vi "tm424_triggermodes.vi"() -> ()   [LabVIEW 2021]
panel:
  in  "Times":i32=1
  in  "Active":i32(ring)=1 items=["Edge"=1, "Level"=2, "Sync Readout"=3, "Point"=4]
  in  "External Options":cluster{"Polarity":i32, "Delay":dbl}={"Polarity"=1, "Delay"=0.0} {"Polarity" items=["Negative"=1, "Positive"=2]}
  in  "Source":i32(ring)=1 items=["Internal"=1, "External"=2, "Software"=3, "Master Pulse"=4]
  out "Timestamp":dbl
  out "Image":u16[][](graph)
  out "Frames Per Second":dbl
  in  "Quit":bool
  out "Error Out":errorcluster {"code" format="%.0x"}
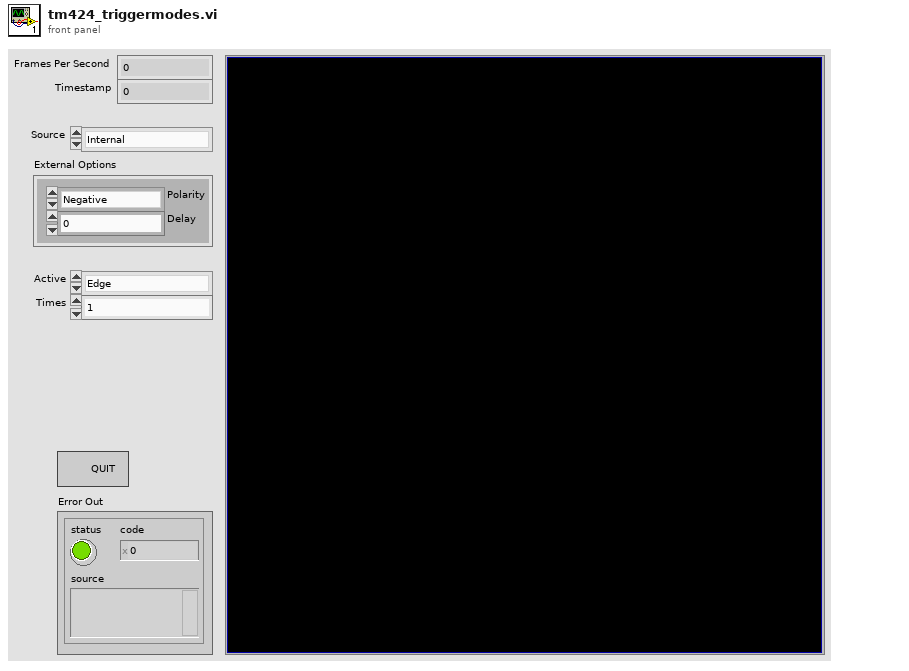
[diagram p1: front panel]
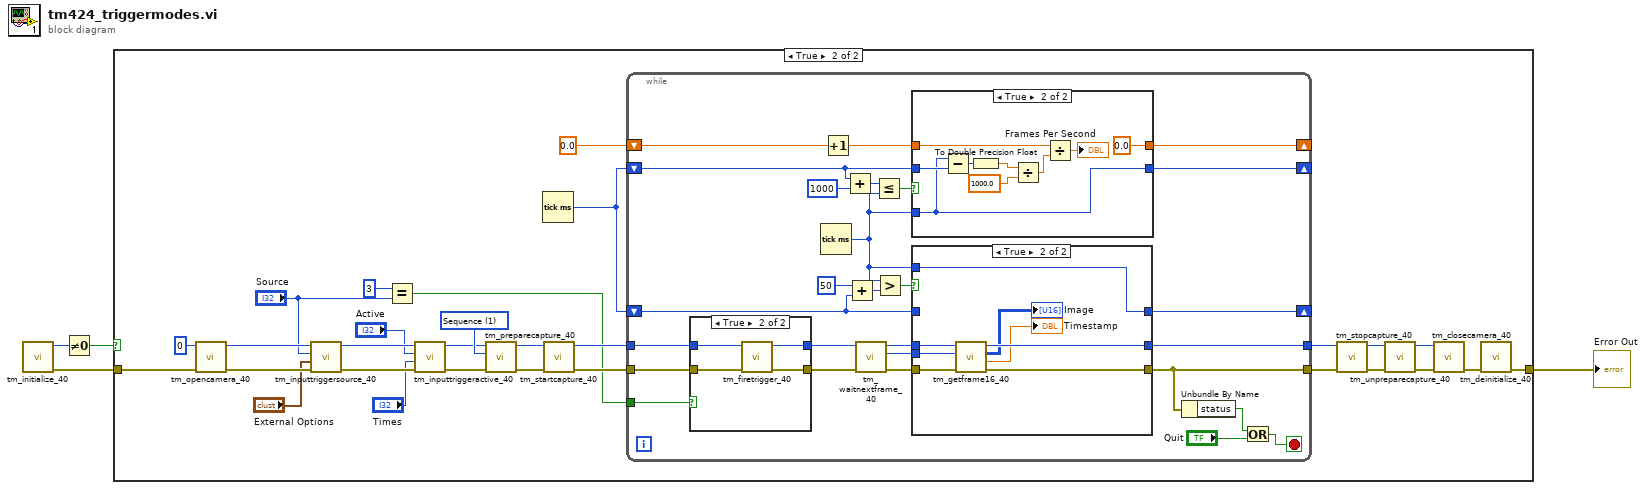
[diagram p0: block diagram]
diagram:
  n1 = call <userlib>:"tm_initialize_40.vi"() -> ("error out"=w2:errorcluster, "Number Of Cameras"=w3:u32)  [unwired: 8 in, 2 out]
  n2 = Not Equal To 0?(x=w3) -> (x != 0?=w4:bool)
  n3 = case shown="True" w4 {
    tunnel: w2 -> [w5 w34]
    tunnel: [w5 w18] -> w1
    frame False {
    }
    frame True {
      w24 = 1 items=["Snap", "Sequence"] ("Capture mode")
      n4 = call <userlib>:"tm_opencamera_40.vi"("error in (no error)"=w34, "Camera Index"=u32 0) -> ("error out"=w17:errorcluster, "Handle out"=w16:u32)  [unwired: 7 in, 1 out]
      n5 = call <userlib>:"tm_inputtriggersource_40.vi"("error in (no error)"=w17, "External Options"="External Options", "Source"="Source", "Handle in"=w16) -> ("error out"=w14:errorcluster, "Handle out"=w15:u32)  [unwired: 6 in]
      n6 = Equal?(x=3, y="Source") -> (x = y?=w6:bool)
      n7 = call <userlib>:"tm_inputtriggeractive_40.vi"("error in (no error)"=w14, "Times"="Times", "Active"="Active", "Handle in"=w15) -> ("error out"=w9:errorcluster, "Handle out"=w10:u32)  [unwired: 6 in]
      n8 = call <userlib>:"tm_preparecapture_40.vi"("error in (no error)"=w9, "Capture mode"=w24, "Handle in"=w10) -> ("error out"=w22:errorcluster, "Handle out"=w23:u32)  [unwired: 5 in, 2 out]
      n9 = Tick Count (ms)() -> (millisecond timer value=w20:u32)
      n10 = call <userlib>:"tm_startcapture_40.vi"("error in (no error)"=w22, "Handle in"=w23) -> ("error out"=w25:errorcluster, "Handle out"=w26:u32)  [unwired: 8 in]
      n11 = while {
        tunnel: [w42] -> w29
        tunnel: [w43] -> w30
        tunnel: w26 -> [w38]
        tunnel: w25 -> [w39]
        shift-right: [w58] -> _
        shift-left: w20 -> [w55]
        shift-right: [w59] -> _
        shift-left: 0.0 -> [w52]
        shift-right: [w41] -> _
        shift-left: w20 -> [w44]
        tunnel: w6 -> [w35]
        stop <- w40 stop-if-true
        n12 = case shown="True" w35 {
          tunnel: w39 -> [w62 w66]
          tunnel: w38 -> [w63 w67]
          tunnel: [w62 w65] -> w36
          tunnel: [w63 w64] -> w37
          frame False {
          }
          frame True {
            n13 = call <userlib>:"tm_firetrigger_40.vi"("error in (no error)"=w66, "Handle in"=w67) -> ("error out"=w65:errorcluster, "Handle out"=w64:u32)  [unwired: 8 in]
          }
        }
        n14 = Tick Count (ms)() -> (millisecond timer value=w45:u32)
        n15 = Increment(x=w52) -> (x+1=w53:dbl)
        n16 = Add(x=w55, y=u32 1000) -> (x+y=w57:u32)
        n17 = Add(x=u32 50, y=w44) -> (x+y=w47:u32)
        n18 = call <userlib>:"tm_waitnextframe_40.vi"("error in (no error)"=w36, "Handle in"=w37) -> ("error out"=w50:errorcluster, "Frame Index"=w49:i32, "Handle out"=w51:u32)  [unwired: 6 in, 1 out]
        n19 = Less Or Equal?(x=w57, y=w45) -> (x <= y?=w54:bool)
        n20 = Greater?(x=w45, y=w47) -> (0:w46:bool)
        n21 = case shown="True" w54 {
          tunnel: w55 -> [w80 w83]
          tunnel: [w80 w81] -> w58
          tunnel: w53 -> [w79 w87]
          tunnel: w45 -> [_ w81]
          tunnel: [w79 0.0] -> w59
          frame False {
          }
          frame True {
            n22 = Subtract(x=w81, y=w83) -> (x-y=w82:u32)
            n23 = To Double Precision Float(number=w82) -> (double precision float=w89:dbl)
            n24 = Divide(x=w89, y=1000.0) -> (x/y=w86:dbl)
            n25 = Divide(x=w87, y=w86) -> (x/y=→"Frames Per Second":dbl)
          }
        }
        n26 = case shown="True" w46 {
          tunnel: w51 -> [w70 w78]
          tunnel: w50 -> [w69 w77]
          tunnel: w49 -> [_ w71]
          tunnel: w44 -> [w68 _]
          tunnel: w45 -> [_ w76]
          tunnel: [w70 w74] -> w42
          tunnel: [w69 w75] -> w43
          tunnel: [w68 w76] -> w41
          frame False {
          }
          frame True {
            n27 = call <userlib>:"tm_getframe16_40.vi"("error in (no error)"=w77, "Frame Index"=w71, "Handle in"=w78) -> ("error out"=w75:errorcluster, "Timestamp"=→"Timestamp":dbl, "Data"=→"Image":u16[][], "Handle out"=w74:u32)  [unwired: 5 in]
          }
        }
        n28 = Unbundle By Name(w43) -> ("status"=w61:bool)
        n29 = Or(x=w61, y="Quit") -> (x .or. y?=w40:bool)
      }
      n30 = call <userlib>:"tm_stopcapture_40.vi"("error in (no error)"=w30, "Handle in"=w29) -> ("error out"=w27:errorcluster, "Handle out"=w28:u32)  [unwired: 8 in]
      n31 = call <userlib>:"tm_unpreparecapture_40.vi"("error in (no error)"=w27, "Handle in"=w28) -> ("error out"=w32:errorcluster, "Handle out"=w31:u32)  [unwired: 8 in]
      n32 = call <userlib>:"tm_closecamera_40.vi"("error in (no error)"=w32, "Handle in"=w31) -> ("error out"=w19:errorcluster)  [unwired: 9 in]
      n33 = call <userlib>:"tm_deinitialize_40.vi"("error in (no error)"=w19) -> ("error out"=w18:errorcluster)  [unwired: 10 in]
    }
  }
  "Error Out" <- w1
